vi "Read Config.vi"(8 "error in (no error)":errorcluster, 11 "GlobalData":T1) -> (0 "error out":errorcluster)   [LabVIEW 2024]
doc: "Load Data from Config File"
uses:
  controls/GlobalData.ctl
  <vilib>/Utility/config.llb/Read Key (String).vi
  <vilib>/Utility/config.llb/NI_LVConfig.lvlib
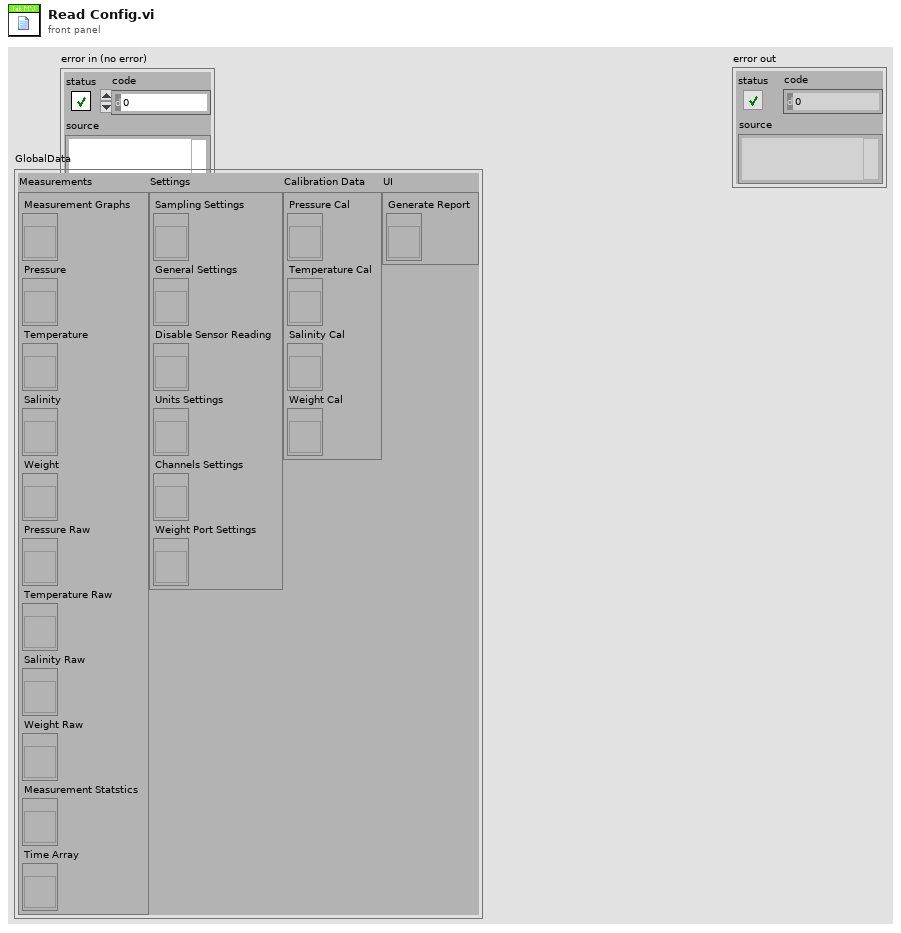
[diagram p1: front panel]
types:
  T1 = typedef "GlobalData.ctl" = cluster{"Measurements":cluster{"Measurement Graphs":refnum<vi>, "Pressure":refnum<vi>, "Temperature":refnum<vi>, "Salinity":refnum<vi>, "Weight":refnum<vi>, "Pressure Raw":refnum<vi>, "Temperature Raw":refnum<vi>, "Salinity Raw":refnum<vi>, "Weight Raw":refnum<vi>, "Measurement Statstics":refnum<vi>, "Time Array":refnum<vi>}, "Settings":cluster{"Sampling Settings":refnum<vi>, "General Settings":refnum<vi>, "Disable Sensor Reading":refnum<vi>, "Units Settings":refnum<vi>, "Channels Settings":refnum<vi>, "Weight Port Settings":refnum<vi>}, "Calibration Data":cluster{"Pressure Cal":refnum<vi>, "Temperature Cal":refnum<vi>, "Salinity Cal":refnum<vi>, "Weight Cal":refnum<vi>}, "UI":cluster{"Generate Report":refnum<vi>}}
  T2 = typedef "NI_LVConfig.lvlib/Config Data RefNum.ctl" = refnum<k1>
  T3 = cluster{"Pressure":cluster{"Physical Channel":tag, "Min Voltage":dbl, "Max Voltage ":dbl, "Terminal Configuration":i32}, "Temperature":cluster{"Physical Channel":tag, "Min Current (mA)":dbl, "Max Current (mA)":dbl, "Terminal Configuration":i32}, "Sallinity":cluster{"Physical Channel":tag, "Min Current (mA)":dbl, "Max Current (mA)":dbl, "Terminal Configuration":i32}}
  T4 = typedef "Serial - Settings.ctl" = cluster{"baud rate":u32, "data bits":u16, "parity":enum16{"None", "Odd", "Even", "Mark", "Space"}, "stop bits":u16, "flow control":u16}
  T5 = cluster{"Port Name":refnum<visa-resource-name>, "Port Settings":T4}
  T6 = cluster{"C (Y-Intercept)":dbl, "M (Gradient)":dbl}
  T7 = typedef "Units.ctl" = cluster{"Pressure":enum16{"PSI", "Bar", "atm", "Pa"}, "Temperature":enum16{"C", "K", "F"}, "Salinity":enum16{"ppm", "ppt", "PSU"}, "Weight":enum16{"Kg", "g", "oz", "ib"}}
  T8 = cluster{"Measurement Statstics":bool, "Logging Type":enum16{"Disable Log", "TDMS", "CSV"}}
  T9 = cluster{"Reading Time (ms)":u64, "Graph Time ":u16}
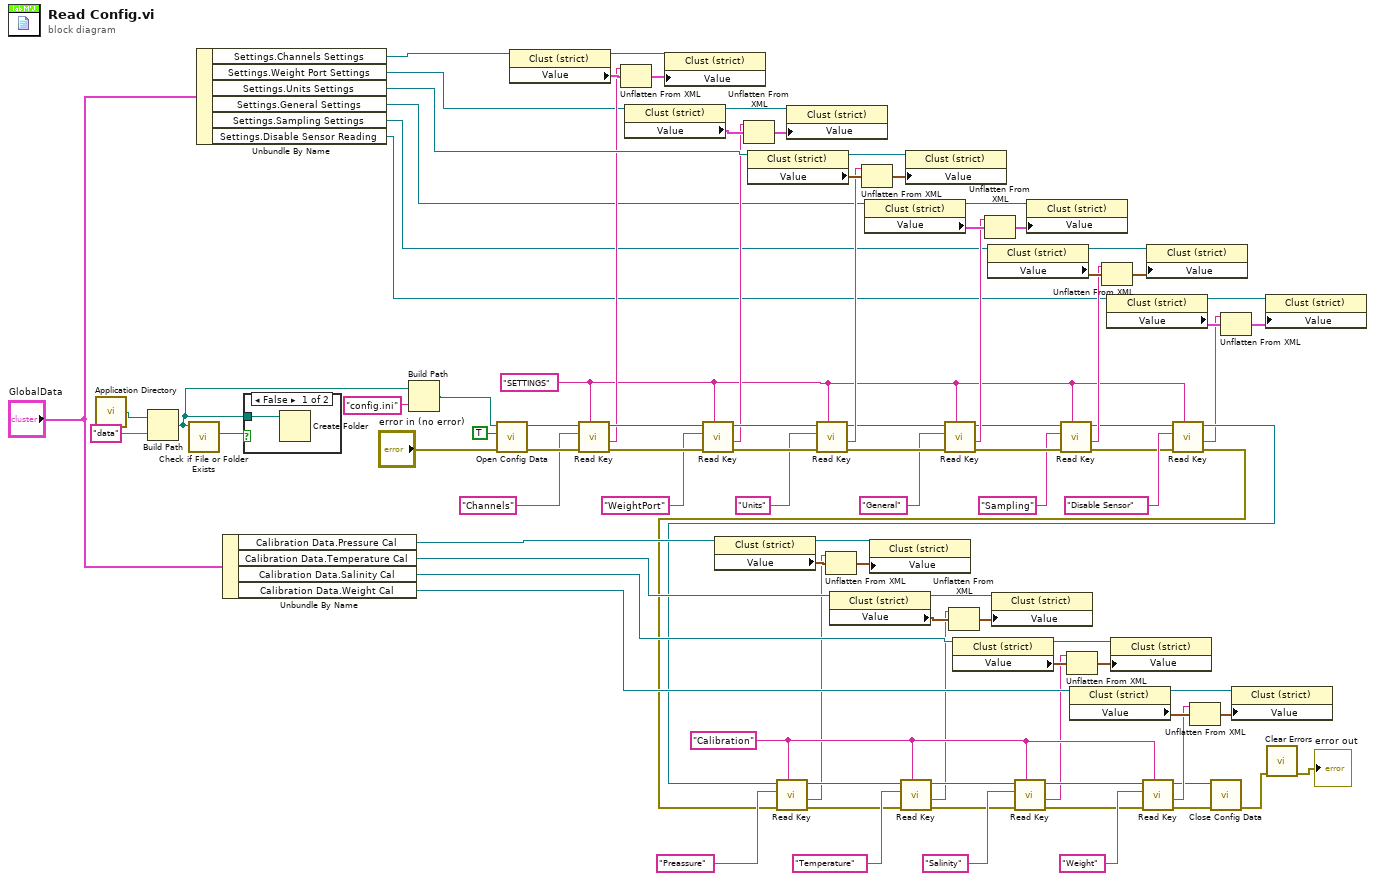
[diagram p0: block diagram]
diagram:
  w53 = "Calibration" ("section")
  w11 = "SETTINGS" ("section")
  n1 = call <vilib>:"Application Directory.vi"() -> ("Application Directory"=w4:path)
  n2 = Build Path(base path=w4, name or relative path="data") -> (appended path=w2:path)
  n3 = call <vilib>:"Check if File or Folder Exists.vi"("path"=w2) -> ("file or folder exists?"=w3:bool)  [unwired: 8 in, 2 out]
  n4 = Unbundle By Name("GlobalData") -> ("Settings.Channels Settings"=w61:refnum<vi>, "Settings.Weight Port Settings"=w54:refnum<vi>, "Settings.Units Settings"=w89:refnum<vi>, "Settings.General Settings"=w73:refnum<vi>, "Settings.Sampling Settings"=w57:refnum<vi>, "Settings.Disable Sensor Reading"=w18:refnum<vi>)
  n5 = Unbundle By Name("GlobalData") -> ("Calibration Data.Pressure Cal"=w30:refnum<vi>, "Calibration Data.Temperature Cal"=w29:refnum<vi>, "Calibration Data.Salinity Cal"=w28:refnum<vi>, "Calibration Data.Weight Cal"=w27:refnum<vi>)
  n6 = case shown="False" w3 {
    tunnel: w2 -> [w96 _]
    frame False {
      n7 = Create Folder(path (use dialog)=w96) -> ()  [unwired: 2 in, 3 out]
    }
    frame True {
    }
  }
  n8 = Build Path(base path=w2, name or relative path="config.ini") -> (appended path=w1:path)
  n9 = call <vilib>:"Open Config Data.vi"("error in (no error)"="error in (no error)", "create file if necessary (T)"=TRUE, "configuration file path"=w1) -> ("error out"=w93:errorcluster, "refnum"=w95:T2)  [unwired: 6 in, 1 out]
  n10 = property class="Clust (strict)"(reference=w61) -> (reference out=w86:refnum<vi>, "Value"=w88:T3)  [unwired: 1 in, 1 out]
  n11 = call-poly <vilib>:"Read Key.vi"("section"=w11, "error in (no error)"=w93, "key"="Channels", "refnum"=w95) -> ("error out"=w92:errorcluster, "value"=w87:string, "refnum out"=w94:T2)  [unwired: 4 in, 1 out]
  n12 = Unflatten From XML(xml string=w87, type=w88) -> (value=w85:T3)  [unwired: 1 in, 1 out]
  n13 = property class="Clust (strict)"(reference=w54) -> (reference out=w82:refnum<vi>, "Value"=w84:T5)  [unwired: 1 in, 1 out]
  n14 = property class="Clust (strict)"(reference=w86, "Value"=w85) -> ()  [unwired: 1 in, 2 out]
  n15 = call-poly <vilib>:"Read Key.vi"("section"=w11, "error in (no error)"=w92, "key"="WeightPort", "refnum"=w94) -> ("error out"=w71:errorcluster, "value"=w83:string, "refnum out"=w90:T2)  [unwired: 4 in, 1 out]
  n16 = property class="Clust (strict)"(reference=w30) -> (reference out=w41:refnum<vi>, "Value"=w42:T6)  [unwired: 1 in, 1 out]
  n17 = Unflatten From XML(xml string=w83, type=w84) -> (value=w81:T5)  [unwired: 1 in, 1 out]
  n18 = property class="Clust (strict)"(reference=w89) -> (reference out=w78:refnum<vi>, "Value"=w80:T7)  [unwired: 1 in, 1 out]
  n19 = property class="Clust (strict)"(reference=w82, "Value"=w81) -> ()  [unwired: 1 in, 2 out]
  n20 = call-poly <vilib>:"Read Key.vi"("section"=w11, "error in (no error)"=w71, "key"="Units", "refnum"=w90) -> ("error out"=w70:errorcluster, "value"=w79:string, "refnum out"=w72:T2)  [unwired: 4 in, 1 out]
  n21 = property class="Clust (strict)"(reference=w29) -> (reference out=w38:refnum<vi>, "Value"=w39:T6)  [unwired: 1 in, 1 out]
  n22 = Unflatten From XML(xml string=w79, type=w80) -> (value=w77:T7)  [unwired: 1 in, 1 out]
  n23 = property class="Clust (strict)"(reference=w73) -> (reference out=w75:refnum<vi>, "Value"=w74:T8)  [unwired: 1 in, 1 out]
  n24 = property class="Clust (strict)"(reference=w78, "Value"=w77) -> ()  [unwired: 1 in, 2 out]
  n25 = call-poly <vilib>:"Read Key.vi"("section"=w11, "error in (no error)"=w70, "key"="General", "refnum"=w72) -> ("error out"=w67:errorcluster, "value"=w69:string, "refnum out"=w68:T2)  [unwired: 4 in, 1 out]
  n26 = property class="Clust (strict)"(reference=w28) -> (reference out=w35:refnum<vi>, "Value"=w36:T6)  [unwired: 1 in, 1 out]
  n27 = Unflatten From XML(xml string=w69, type=w74) -> (value=w76:T8)  [unwired: 1 in, 1 out]
  n28 = property class="Clust (strict)"(reference=w57) -> (reference out=w55:refnum<vi>, "Value"=w65:T9)  [unwired: 1 in, 1 out]
  n29 = property class="Clust (strict)"(reference=w75, "Value"=w76) -> ()  [unwired: 1 in, 2 out]
  n30 = call-poly <vilib>:"Read Key.vi"("section"=w11, "error in (no error)"=w67, "key"="Sampling", "refnum"=w68) -> ("error out"=w15:errorcluster, "value"=w64:string, "refnum out"=w12:T2)  [unwired: 4 in, 1 out]
  n31 = property class="Clust (strict)"(reference=w27) -> (reference out=w32:refnum<vi>, "Value"=w31:T6)  [unwired: 1 in, 1 out]
  n32 = Unflatten From XML(xml string=w64, type=w65) -> (value=w66:T9)  [unwired: 1 in, 1 out]
  n33 = property class="Clust (strict)"(reference=w18) -> (reference out=w17:refnum<vi>, "Value"=w20:cluster{"Daq":bool, "RS232":bool})  [unwired: 1 in, 1 out]
  n34 = property class="Clust (strict)"(reference=w55, "Value"=w66) -> ()  [unwired: 1 in, 2 out]
  n35 = call-poly <vilib>:"Read Key.vi"("section"=w11, "error in (no error)"=w15, "key"="Disable Sensor", "refnum"=w12) -> ("error out"=w14:errorcluster, "value"=w10:string, "refnum out"=w13:T2)  [unwired: 4 in, 1 out]
  n36 = call-poly <vilib>:"Read Key.vi"("section"=w53, "error in (no error)"=w14, "key"="Preassure", "refnum"=w13) -> ("error out"=w44:errorcluster, "value"=w26:string, "refnum out"=w43:T2)  [unwired: 4 in, 1 out]
  n37 = Unflatten From XML(xml string=w26, type=w42) -> (value=w40:T6)  [unwired: 1 in, 1 out]
  n38 = property class="Clust (strict)"(reference=w41, "Value"=w40) -> ()  [unwired: 1 in, 2 out]
  n39 = call-poly <vilib>:"Read Key.vi"("section"=w53, "error in (no error)"=w44, "key"="Temperature", "refnum"=w43) -> ("error out"=w47:errorcluster, "value"=w25:string, "refnum out"=w45:T2)  [unwired: 4 in, 1 out]
  n40 = Unflatten From XML(xml string=w25, type=w39) -> (value=w37:T6)  [unwired: 1 in, 1 out]
  n41 = property class="Clust (strict)"(reference=w38, "Value"=w37) -> ()  [unwired: 1 in, 2 out]
  n42 = call-poly <vilib>:"Read Key.vi"("section"=w53, "error in (no error)"=w47, "key"="Salinity", "refnum"=w45) -> ("error out"=w48:errorcluster, "value"=w24:string, "refnum out"=w46:T2)  [unwired: 4 in, 1 out]
  n43 = Unflatten From XML(xml string=w24, type=w36) -> (value=w34:T6)  [unwired: 1 in, 1 out]
  n44 = property class="Clust (strict)"(reference=w35, "Value"=w34) -> ()  [unwired: 1 in, 2 out]
  n45 = call-poly <vilib>:"Read Key.vi"("section"=w53, "error in (no error)"=w48, "key"="Weight", "refnum"=w46) -> ("error out"=w21:errorcluster, "value"=w23:string, "refnum out"=w22:T2)  [unwired: 4 in, 1 out]
  n46 = Unflatten From XML(xml string=w23, type=w31) -> (value=w33:T6)  [unwired: 1 in, 1 out]
  n47 = call <vilib>:"Close Config Data.vi"("error in (no error)"=w21, "refnum"=w22) -> ("error out"=w8:errorcluster)  [unwired: 8 in, 1 out]
  n48 = Unflatten From XML(xml string=w10, type=w20) -> (value=w19:cluster{"Daq":bool, "RS232":bool})  [unwired: 1 in, 1 out]
  n49 = property class="Clust (strict)"(reference=w32, "Value"=w33) -> ()  [unwired: 1 in, 2 out]
  n50 = property class="Clust (strict)"(reference=w17, "Value"=w19) -> ()  [unwired: 1 in, 2 out]
  n51 = call <vilib>:"Clear Errors.vi"("error in (no error)"=w8) -> ("error out"=→"error out":errorcluster)  [unwired: 5 in, 1 out]
